vi "Fetch.vi"(8 "error in (no error)":errorcluster, 10 "Message in":refnum<class "FetchMessage.lvclass">, 11 "MeritFactor in":refnum<class "MeritFactor.lvclass">) -> (0 "error out":errorcluster, 3 "MeritFactor out":refnum<class "MeritFactor.lvclass">)   [LabVIEW 2012, in "MeritFactor.lvclass"]
doc: "The fetch method processes the command 'fetch'. \n\nThe command 'fetch' is used for receiving various forms of data."
uses:
  MeritFactor.lvclass
  <vilib>/Distrio/Murmex/FetchMessage/FetchMessage.lvclass
  <vilib>/Distrio/Murmex/Murmex/Murmex.lvclass
  <vilib>/vision/Image Controls.llb/IMAQ Image.ctl
  MeritFactor.lvclass/MeritFactor.ctl
panel:
  # "This method is called when the FETCH\ntrigger is sent. \n\nOverride this method when your component needs to\nrespond to this trigger. \n\nCall parent for proper implementation"
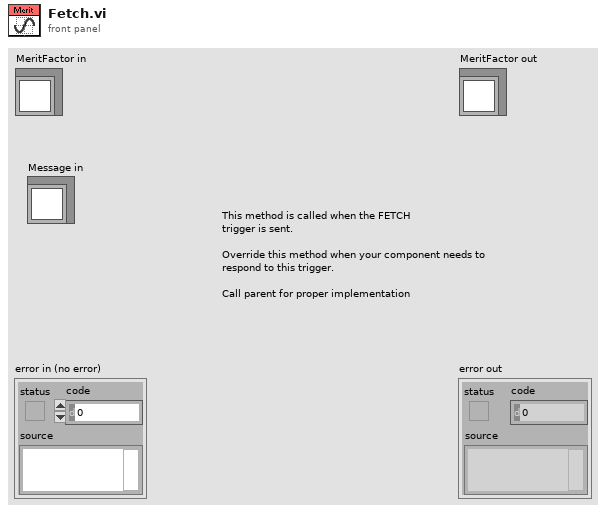
[diagram p1: front panel]
types:
  T1 = typedef "IMAQ Image.ctl" = refnum<image>
  T2 = typedef "Murmex.lvlib/FetchMessage.lvclass/Channel data cluster.ctl" = cluster{"channel id":i32, "data UInt8":u8[], "data type":T3, "dimensions":i32[], "physical units":T4[], "waveform dt":dbl, "waveform":T5}
  T3 = typedef "Murmex.lvlib/Murmex.lvclass/data_type_enum.ctl" = enum16{"Float128", "Float64", "Float32", "Int64", "Int32", "Int16", "Int8", "UInt64", "UInt32", "UInt16", "UInt8", "Boolean", "String"}
  T4 = typedef "Physical Units__ogtk.ctl" = cluster{"Base Units":enum16{"radian", "steradian", "second", "meter", "kilogram", "ampere", "kelvin", "mole", "candela"}, "Exponent":i16}
  T5 = typedef "Murmex.lvlib/Murmex.lvclass/waveform_type_enum.ctl" = enum16{"no waveform", "analog", "digital"}
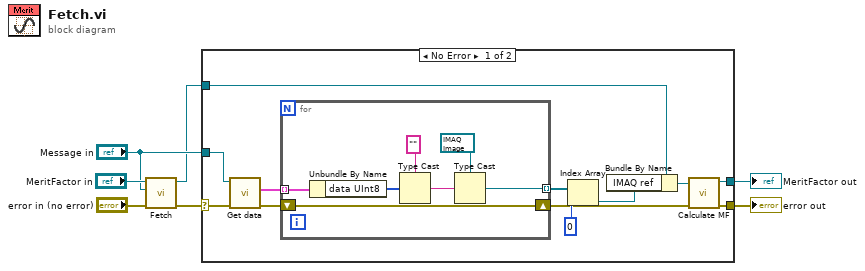
[diagram p0: block diagram]
diagram:
  n1 = call-parent "Fetch.vi"("error in (no error)"="error in (no error)", "Message in"="Message in", "Murmex in"="MeritFactor in") -> ("error out"=w5:errorcluster, "Murmex out"=w3:refnum<class "MeritFactor.lvclass">)  [unwired: 7 in]
  n2 = case shown="No Error" w5 {
    selector: w5 -> [w19 w27]
    tunnel: "Message in" -> [w16 _]
    tunnel: w3 -> [w10 w28]
    tunnel: [w12 w28] -> w2
    tunnel: [w11 w27] -> w1
    frame No Error {
      n3 = call <vilib>:"Get data.vi"("error in (no error)"=w19, "FetchMessage.lvclass"=w16) -> ("error out"=w18:errorcluster, "data (channels)"=w17:T2[])  [unwired: 7 in, 1 out]
      n4 = for {
        shift-right: [w25] -> w13
        shift-left: w18 -> [w25]
        tunnel: w17 -> [w26] mode=indexing
        tunnel: [w20] -> w15 mode=indexing
        n5 = Unbundle By Name(w26) -> ("data UInt8"=w24:u8[])
        n6 = Type Cast(type="", x=w24) -> (*(type *) &x=w22:string)
        n7 = Type Cast(type=T1 refnum ("Image Dst Out"), x=w22) -> (*(type *) &x=w20:T1)
      }
      n8 = Index Array(array=w15, index=0 ("index (row)")) -> (element=w9:T1)
      n9 = Bundle By Name(cluster=w10, "IMAQ ref"=w9) -> (w8:refnum<class "MeritFactor.lvclass">)
      n10 = call-dynamic "Calculate MF.vi"("error in (no error)"=w13, "MeritFactor in"=w8) -> ("error out"=w11:errorcluster, "MeritFactor out"=w12:refnum<class "MeritFactor.lvclass">)  [unwired: 8 in]
    }
    frame Error {
    }
  }
  "error out" <- w1
  "MeritFactor out" <- w2
